vi "Auto External Data Log Range.vi"(7 "External Data Log Auto Range (False)":bool, 8 "error in (no error)":errorcluster {"code" format="%.0x"}, 9 "External Data Log Type (1: Voltage)":i32(ring)=1 items=["Voltage"=1, "Current"=0], 10 "Channel Name (1)":string="1", 11 "VISA resource name":refnum<visa-resource-name>) -> (0 "error out":errorcluster {"code" format="%.0x"}, 3 "VISA resource name out":refnum<visa-resource-name>)   [LabVIEW 2016, in "Agilent N6700 Series.lvlib"]
doc: "Enables or disables the external datalog measurement autoranging.\n\n<b>Notes:</b>\n(1) This VI only applies to N678xA modules.\n(2) When enabled, this VI overrides the setting in <B>Configure External Log Range.vi</B>."
uses:
  <instrlib>/Agilent N6700 Series/Agilent N6700 Series.lvlib
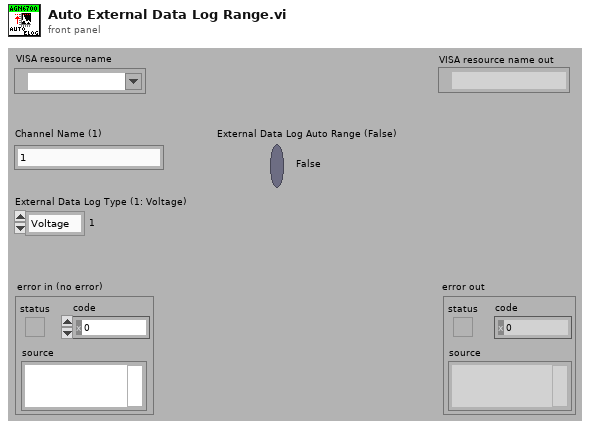
[diagram p1: front panel]
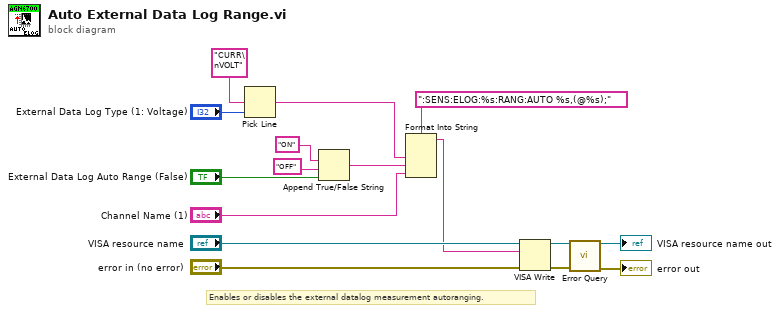
[diagram p0: block diagram]
diagram:
  # "Enables or disables the external datalog measurement autoranging."
  n1 = Pick Line(multi-line string="CURR\nVOLT", line index="External Data Log Type (1: Voltage)") -> (output string=w7:string)  [unwired: 1 in]
  n2 = Append True/False String(1:"External Data Log Auto Range (False)", 2:"OFF", 3:"ON") -> (0:w3:string)  [unwired: 1 in]
  n3 = Format Into String(format string=":SENS:ELOG:%s:RANG:AUTO %s,(@%s);", w7, w3, "Channel Name (1)") -> (resulting string=w1:string)  [unwired: 2 in, 1 out]
  n4 = VISA Write(VISA resource name="VISA resource name", write buffer=w1, error in (no error)="error in (no error)") -> (VISA resource name out=w12:refnum<visa-resource-name>, error out=w11:errorcluster)  [unwired: 1 out]
  n5 = call <instrlib>:"Error Query.vi"("VISA resource name"=w12, "error in (no error)"=w11) -> ("VISA resource name out"=→"VISA resource name out":refnum<visa-resource-name>, "error out"=→"error out":errorcluster)  [unwired: 10 in, 2 out]
